vi "S2DS_Master Edit.vi"(7 "External control settings":i32[](array[numeric]), 8 "error in":errorcluster, 9 "Data saving info":T1={"File path"=path "", "Header"="", "File name"="", "False channel"=[], "Channel names"=[], "Buffer size"=0, "Format"="%.6f"}, 10 "All channel parameters":T2 {"Scan parameters"."Y data taking" items=["in both direction", "in up direction only", "in down direction only"]; "Scan parameters"."X data taking" items=["in both direction", "in up direction only", "in down direction only"]}, 11 "Instrument Info (in)":T11) -> (0 "error out":errorcluster, 1 "Data saving info (out)":T1={"File path"=path "", "Header"="", "File name"="", "False channel"=[], "Channel names"=[], "Buffer size"=0, "Format"="%.6f"}, 2 "All channel parameters (out)":T2 {"Scan parameters"."Y data taking" items=["in both direction", "in up direction only", "in down direction only"]; "Scan parameters"."X data taking" items=["in both direction", "in up direction only", "in down direction only"]}, 3 "Instrument Info (out)":T11, 4 "Update instruction":i32[](array[numeric]), 5 "External control settings out":i32[](array[numeric]))   [LabVIEW 2025]
uses:
  TYPE DEFS/S2DS_Instrument Info.ctl
  TYPE DEFS/S2DS_Instrument parameters.ctl
  TYPE DEFS/S2DS_All Channel Parameters.ctl
  TYPE DEFS/S2DS_WC info.ctl
  TYPE DEFS/S2DS_Single WC info.ctl
  TYPE DEFS/S2DS_RC info.ctl
  TYPE DEFS/S2DS_Single RC info.ctl
  TYPE DEFS/S2DS_DAC info new.ctl
  TYPE DEFS/S2DS_Single DC info.ctl
  TYPE DEFS/S2DS_Array Inst Info.ctl
  TYPE DEFS/S2DS_Sweep Info.ctl
  TYPE DEFS/S2DS_Data saving info.ctl
panel:
  in  "Data save info":bool
  in  "Edit DC?":bool
  in  "External control settings":bool
  in  "Sweep channel":bool
  in  "Save to file":bool
  in  "Load from file":bool
  in  "Add script file?":bool
  in  "Edit Instrument?":bool
  in  "Edit RC?":bool
  in  "Edit WC?":bool
  in  "OK 2":bool
  # "SETTINGS..."
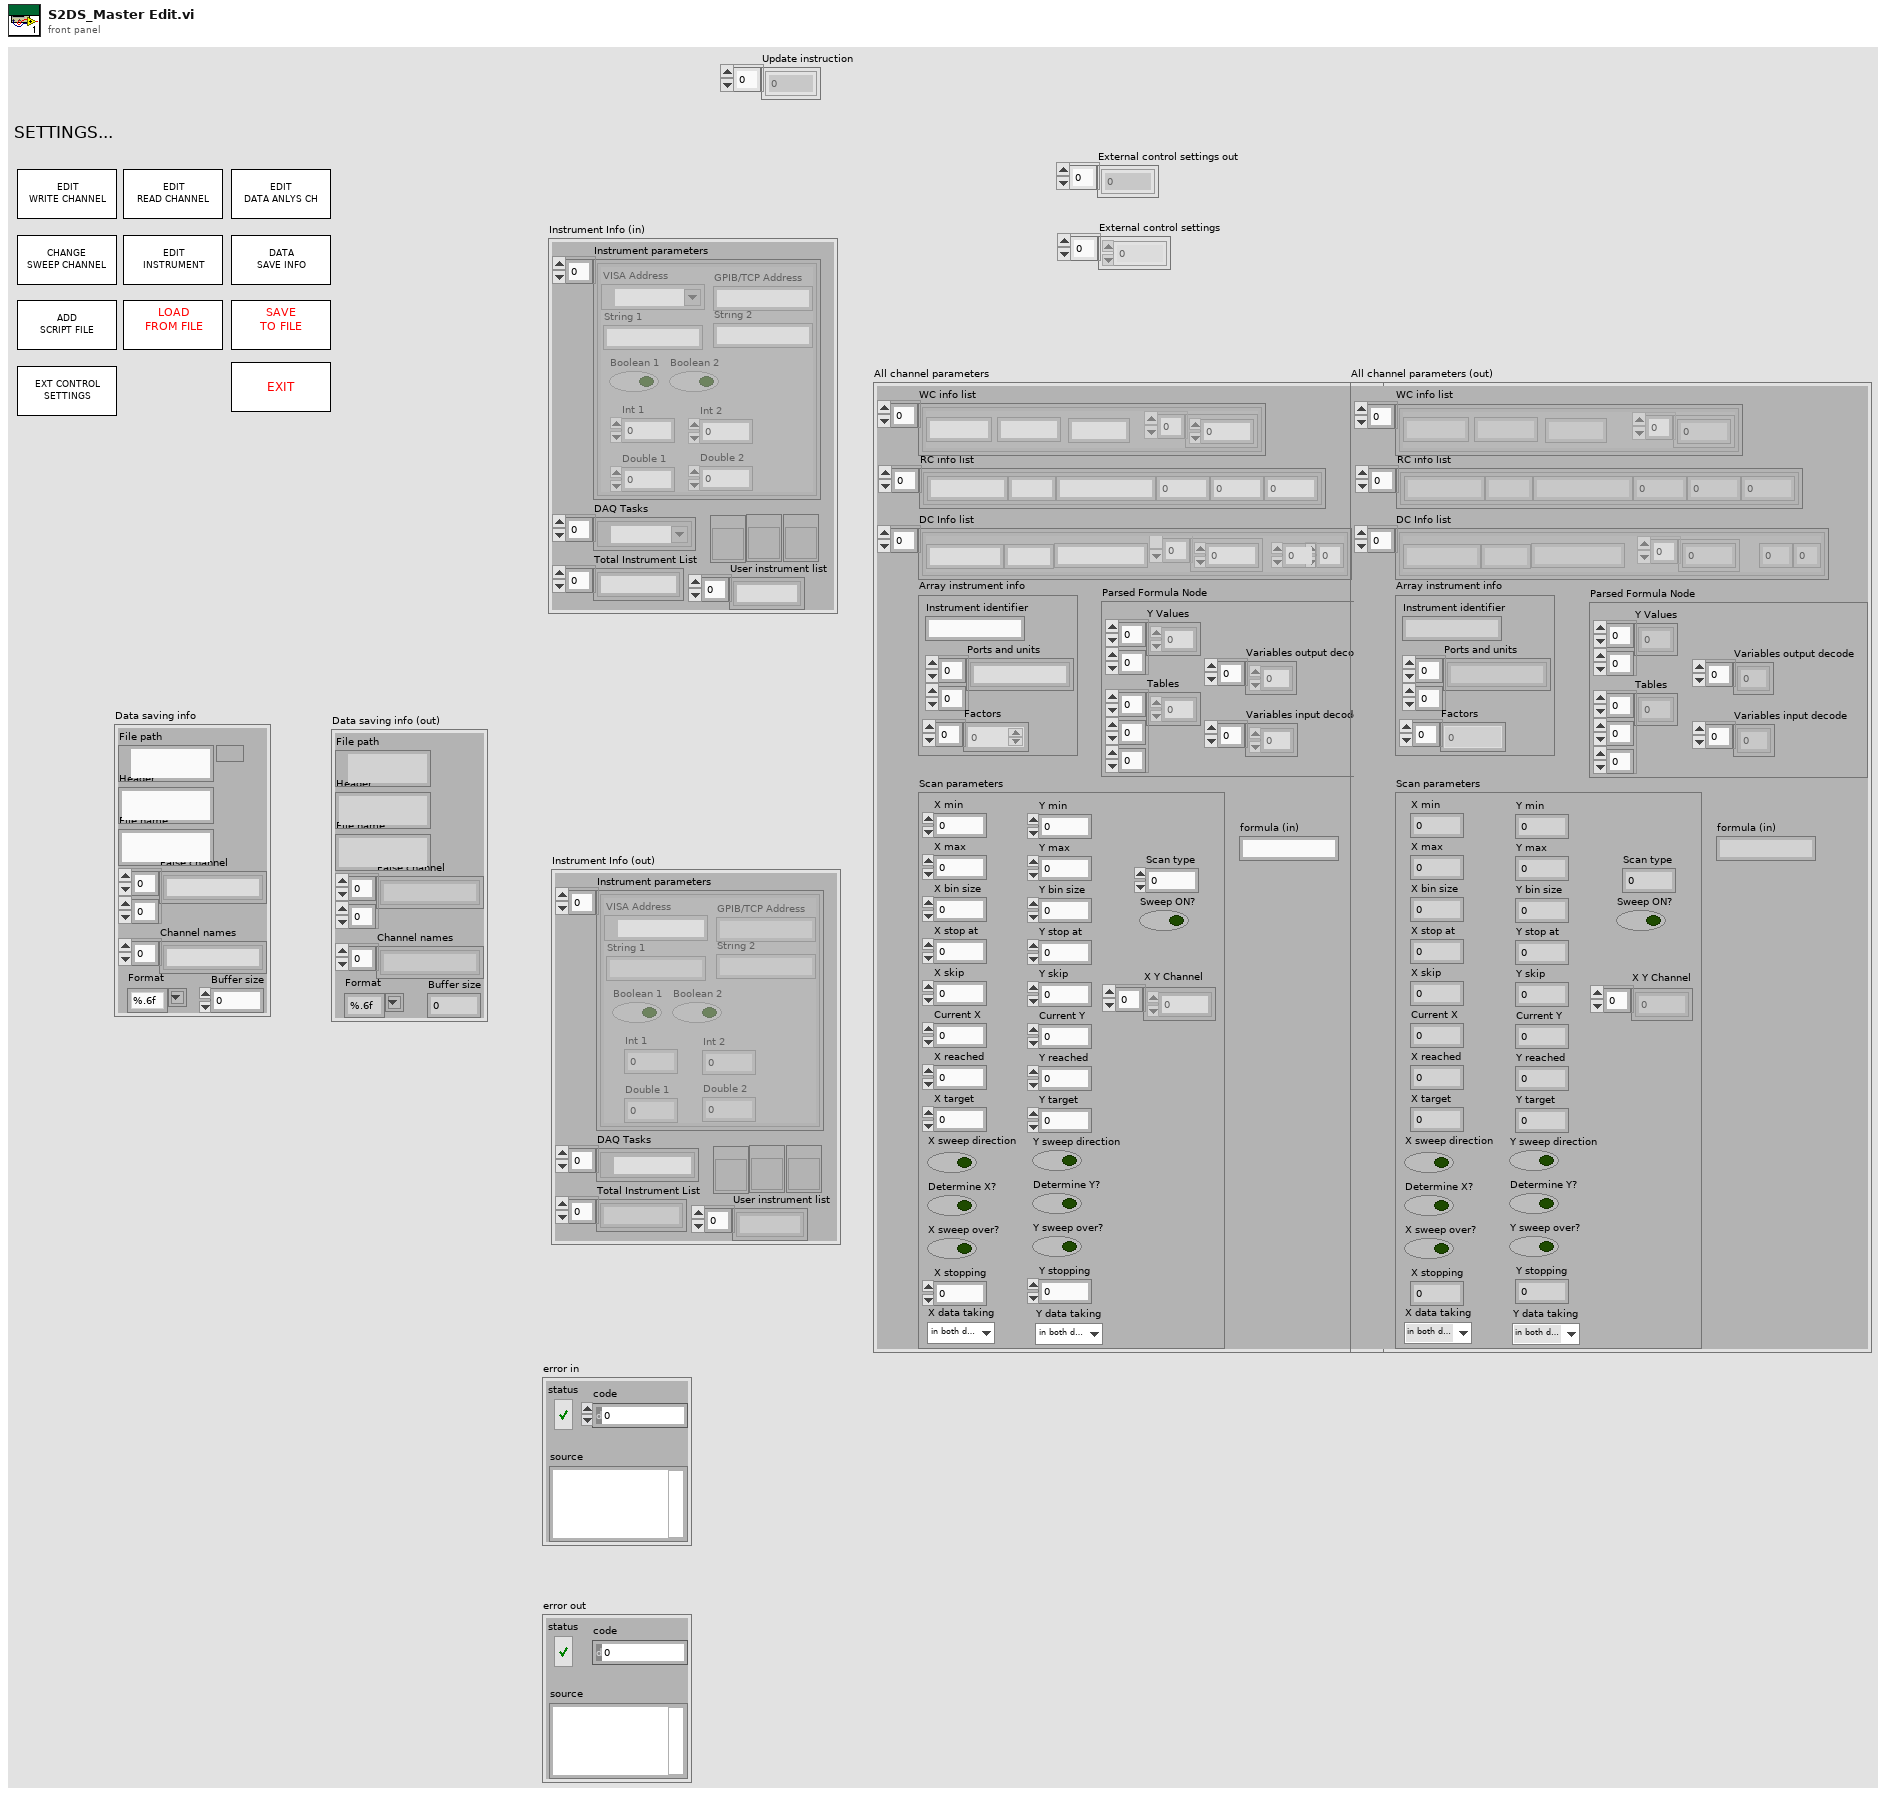
[diagram p1: front panel]
types:
  T1 = typedef "S2DS_Data saving info.ctl" = cluster{"File path":path, "Header":string, "File name":string, "False channel":string[][], "Channel names":string[], "Buffer size":i32, "Format":string}
  T2 = typedef "S2DS_All Channel Parameters.ctl" = cluster{"WC info list":T3, "RC info list":T5, "DC Info list":T7, "Array instrument info":T9, "Scan parameters":T10, "Parsed Formula Node":cluster{"Y Values":dbl[][], "Tables":i32[][][], "Variables input decode":i32[], "Variables output decode":i32[]}, "formula (in)":string}
  T3 = typedef "S2DS_WC info.ctl" = T4[]
  T4 = typedef "S2DS_Single WC info.ctl" = cluster{"Instrument identifier":string, "Write channel parameters":dbl[], "Name":string, "Unit":string}
  T5 = typedef "S2DS_RC info.ctl" = T6[]
  T6 = typedef "S2DS_Single RC info.ctl" = cluster{"Instrument identifier":string, "Factor":dbl, "Averaging":i32, "Wait (ms)":i32, "Unit":string, "Name":string}
  T7 = typedef "S2DS_DAC info new.ctl" = T8[]
  T8 = typedef "S2DS_Single DC info.ctl" = cluster{"Operation identifier":string, "DC parameters":dbl[], "U":i32, "V":i32, "Name":string, "Unit":string}
  T9 = typedef "S2DS_Array Inst Info.ctl" = cluster{"Instrument identifier":string, "Ports and units":string[][], "Factors":dbl[]}
  T10 = typedef "S2DS_Sweep Info.ctl" = cluster{"X min":ext, "X max":dbl, "Y min":dbl, "Y max":dbl, "X bin size":dbl, "Y bin size":dbl, "X stop at":dbl, "Y stop at":dbl, "X skip":u64, "Y skip":u64, "Current X":dbl, "Current Y":dbl, "X reached":i32, "Y reached":i32, "X target":dbl, "Y target":dbl, "Sweep ON?":bool, "X sweep direction":bool, "Y sweep direction":bool, "Determine X?":bool, "Determine Y?":bool, "X sweep over?":bool, "Y sweep over?":bool, "Scan type":i32, "X stopping":i32, "Y stopping":i32, "X Y Channel":u16[], "X data taking":u16, "Y data taking":u16}
  T11 = typedef "S2DS_Instrument Info.ctl" = cluster{"Instrument parameters":T12[], "DAQ Tasks":refnum<k21>[], "Total Instrument List":string[], "read inst \nVI Refnum":refnum<vi>, "type specifier Edit instruments VI Refnum":refnum<vi>, "type specifier write instrument VI Refnum (for type only)":refnum<vi>, "User instrument list":string[]}
  T12 = typedef "S2DS_Instrument parameters.ctl" = cluster{"VISA Address":refnum<visa-resource-name>, "GPIB/TCP Address":string, "String 1":string, "String 2":string, "Boolean 1":bool, "Boolean 2":bool, "Int 1":i32, "Int 2":i32, "Double 1":dbl, "Double 2":dbl}
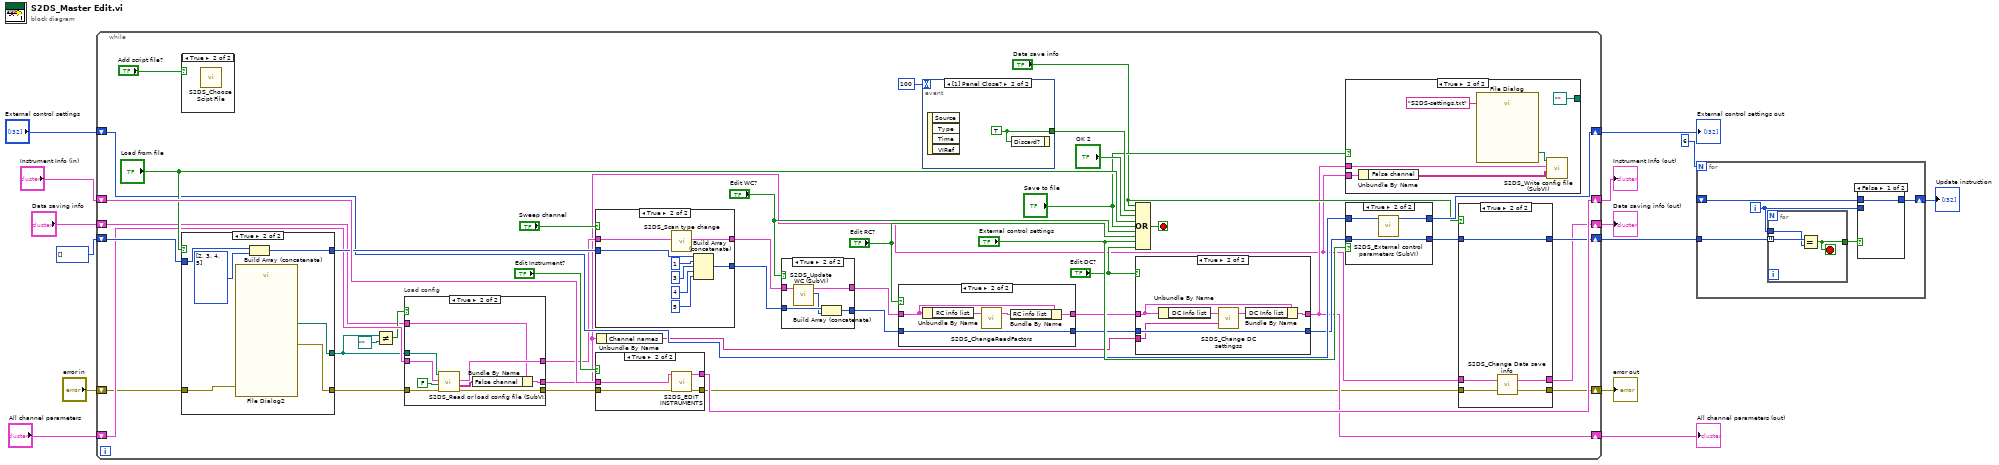
[diagram p0: block diagram]
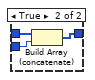
[diagram p2: hidden frame]
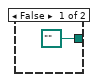
[diagram p8: hidden frame]
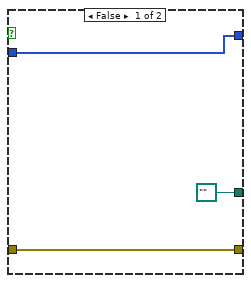
[diagram p9: hidden frame]
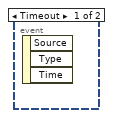
[diagram p14: hidden frame]
diagram:
  n1 = while {
    shift-right: [w20] -> w9
    shift-left: "All channel parameters" -> [w32]
    shift-right: [w52] -> w12
    shift-left: "Instrument Info (in)" -> [w53]
    shift-right: [w18] -> w13
    shift-left: "error in" -> [w29]
    shift-right: [w22] -> w5
    shift-left: i32[] [] -> [w40]
    shift-right: [w21] -> w6
    shift-left: "Data saving info" -> [w17]
    shift-right: [w38] -> w1
    shift-left: "External control settings" -> [w37]
    stop <- w55 stop-if-true
    n2 = case shown="True" "Add script file?" {
      frame False {
      }
      frame True {
        n3 = call "S2DS_Choose Scipt File.vi"() -> ()  [unwired: 12 in]
      }
    }
    n4 = case shown="True" "Load from file" {
      tunnel: [path "" w117] -> w27
      tunnel: [w110 w115] -> w41
      tunnel: w40 -> [w110 w116]
      tunnel: [w109 w113] -> w31
      tunnel: w29 -> [w109 w112]
      frame False {
      }
      frame True {
        n5 = call "File Dialog2"("error in"=w112) -> ("selected path"=w117:path, "error out"=w113:errorcluster)  [unwired: 11 in, 2 out]
        n6 = Build Array (concatenate)(w116, i32[] [2, 3, 4, 5] ("array")) -> (w115:i32[])
      }
    }
    n7 = Not Equal?(x=w27, y=path "") -> (x != y?=w26:bool)
    n8 = case "Load config" shown="True" w26 {
      tunnel: w32 -> [w69 w78]
      tunnel: [w69 w77] -> w25
      tunnel: w31 -> [w68 w76]
      tunnel: [w68 w75] -> w30
      tunnel: w27 -> [_ w74]
      tunnel: [w67 w70] -> w16
      tunnel: w17 -> [w67 w72]
      frame False {
      }
      frame True {
        n9 = call "S2DS_Read or load config file (SubVI).vi"("error in (no error)"=w76, "Update present value?"=FALSE ("Accept target?"), "All channel parameters (in)"=w78, "selected path"=w74) -> ("error out"=w75:errorcluster, "False channel (out)"=w71:string[][], "All channel parameters (out)"=w77:T2)  [unwired: 4 in, 1 out]
        n10 = Bundle By Name(cluster=w72, "False channel"=w71) -> (w70:T1)
      }
    }
    n11 = case shown="True" "Sweep channel" {
      tunnel: w25 -> [w93 w101]
      tunnel: [w93 w100] -> w43
      tunnel: [w92 w97] -> w42
      tunnel: w41 -> [w92 w98]
      frame False {
      }
      frame True {
        n12 = call "S2DS_Scan type change.vi"("All channel parameters"=w101) -> ("All channel parameters (out)"=w100:T2)  [unwired: 10 in]
        n13 = Build Array (concatenate)(w98, 1, 3 ("element"), 4 ("element"), 5 ("element")) -> (w97:i32[])
      }
    }
    n14 = case shown="True" "Edit Instrument?" {
      tunnel: w53 -> [w119 w123]
      tunnel: w30 -> [w118 w122]
      tunnel: [w118 w120] -> w19
      tunnel: [w119 w121] -> w52
      frame False {
      }
      frame True {
        n15 = call "S2DS_EDIT INSTRUMENTS.vi"("error in (no error)"=w122, "Instrument Info (in)"=w123) -> ("error out"=w120:errorcluster, "Instrument Info (out)"=w121:T11)  [unwired: 4 in]
      }
    }
    n16 = Unbundle By Name(w16) -> ("Channel names"=w15:string[])
    n17 = case shown="True" "Edit WC?" {
      tunnel: w43 -> [w132 w135]
      tunnel: [w132 w134] -> w50
      tunnel: [w131 w136] -> w45
      tunnel: w42 -> [w131 w137]
      frame False {
      }
      frame True {
        n18 = call "S2DS_Update WC (SubVI).vi"("All channel parameters (in)"=w135) -> ("Change required"=w133:i32[], "All channel parameters (out)"=w134:T2)  [unwired: 9 in]
        n19 = Build Array (concatenate)(w137, w133) -> (w136:i32[])
      }
    }
    n20 = case shown="True" "Edit RC?" {
      tunnel: w50 -> [w125 w129]
      tunnel: [w125 w127] -> w36
      tunnel: [w124 w126] -> w34
      tunnel: w45 -> [w124 w126]
      frame False {
      }
      frame True {
        n21 = Unbundle By Name(w129) -> ("RC info list"=w130:T5)
        n22 = call "S2DS_ChangeReadFactors.vi"("RC info list (in)"=w130) -> ("RC info list (out)"=w128:T5)  [unwired: 2 in]
        n23 = Bundle By Name(cluster=w129, "RC info list"=w128) -> (w127:T2)
      }
    }
    n24 = event shown="[1] Panel Close?" {
      selector: _ -> [_ _]
      dyn-events: _ -> [_ _]
      timeout: 100 -> [_ _]
      tunnel: [_ w138] -> w57
      event Timeout {
        n25 = event-data() -> ()  [unwired: 1 in, 3 out]
      }
      event Panel Close? {
        w138 = TRUE ("Discard?")
        n26 = event-data() -> ()  [unwired: 1 in, 4 out]
        n27 = event-data("Discard?"=w138) -> ()  [unwired: 1 in, 1 out]
      }
    }
    n28 = Compound Arithmetic op=OR("Data save info", w57, "OK 2", "Load from file", "Save to file", "Edit WC?", "Edit RC?", "External control settings", "Edit DC?") -> (w55:bool)
    n29 = case shown="True" "Edit DC?" {
      tunnel: [w80 w85] -> w20
      tunnel: w36 -> [w80 w86]
      tunnel: [w79 w83] -> w35
      tunnel: w34 -> [w79 w83]
      tunnel: w15 -> [_ w81]
      frame False {
      }
      frame True {
        n30 = Unbundle By Name(w86) -> ("DC Info list"=w82:T7)
        n31 = call "S2DS_Change DC settingss.vi"("Channel names"=w81, "DC Info list"=w82) -> ("DC Info list 2"=w84:T7)  [unwired: 1 in]
        n32 = Bundle By Name(cluster=w86, "DC Info list"=w84) -> (w85:T2)
      }
    }
    n33 = case shown="True" "Save to file" {
      tunnel: [path "" path ""] -> _
      tunnel: w20 -> [_ w107]
      tunnel: w16 -> [_ w104]
      frame False {
      }
      frame True {
        n34 = Unbundle By Name(w104) -> ("False channel"=w103:string[][])
        n35 = call "File Dialog"("default name"="S2DS-settings.txt") -> ("selected path"=w106:path)  [unwired: 11 in, 3 out]
        n36 = call "S2DS_Write config file (SubVI).vi"("False channel"=w103, "All channel parameters"=w107, "file path (use dialog)"=w106) -> ()  [unwired: 7 in, 2 out]
      }
    }
    n37 = case shown="True" "External control settings" {
      tunnel: [w88 w90] -> w38
      tunnel: w37 -> [w88 w91]
      tunnel: [w87 w89] -> w23
      tunnel: w35 -> [w87 w89]
      frame False {
      }
      frame True {
        n38 = call "S2DS_External control parameters (SubVI).vi"("Array in"=w91) -> ("Array out"=w90:i32[])  [unwired: 10 in]
      }
    }
    n39 = case shown="True" "Data save info" {
      tunnel: [w61 w66] -> w22
      tunnel: w23 -> [w61 w66]
      tunnel: [w60 w62] -> w21
      tunnel: w16 -> [w60 w63]
      tunnel: w19 -> [w59 w65]
      tunnel: [w59 w64] -> w18
      frame False {
      }
      frame True {
        n40 = call "S2DS_Change Data save info.vi"("error in (no error)"=w65, "Data saving info"=w63) -> ("error out"=w64:errorcluster, "Data saving info 2"=w62:T1)
      }
    }
  }
  "error out" <- w13
  "Instrument Info (out)" <- w12
  "All channel parameters (out)" <- w9
  "Data saving info (out)" <- w6
  "External control settings out" <- w1
  n41 = for {
    N: 6 -> [_]
    tunnel: w5 -> [w143]
    shift-right: [w141] -> w3
    shift-left: _ -> [w140]
    i -> [w142]
    n42 = for {
      tunnel: w143 -> [w150] mode=indexing
      tunnel: w142 -> [w149]
      tunnel: [w148] -> w139
      stop <- w148 stop-if-true
      n43 = Equal?(x=w150, y=w149) -> (x = y?=w148:bool)
    }
    n44 = case shown="False" w139 {
      tunnel: w142 -> [_ w147]
      tunnel: [w144 w146] -> w141
      tunnel: w140 -> [w144 w145]
      frame False {
      }
      frame True {
        n45 = Build Array (concatenate)(w145, w147) -> (w146:i32[])
      }
    }
  }
  "Update instruction" <- w3
